vi "Handle Error.vi"(7 "Mode":T1(ring), 8 "error in (no error)":errorcluster, 9 "Test Method Name":string, 11 "Test Case Result In":refnum<class "Test Case Result.lvclass">) -> (0 "error out":errorcluster, 3 "Test Case Result Out":refnum<class "Test Case Result.lvclass">)   [LabVIEW 2020, in "Test Case Result.lvclass"]
uses:
  Test Case Result.lvclass
  Test Case Result.lvclass/Test Case Result.ctl
  Method Result/Method Result.lvclass/Method Result.ctl
  <vilib>/Utility/miscctls.llb/LVMapReplaceAction.ctl
  Method Result/Method Result.lvclass
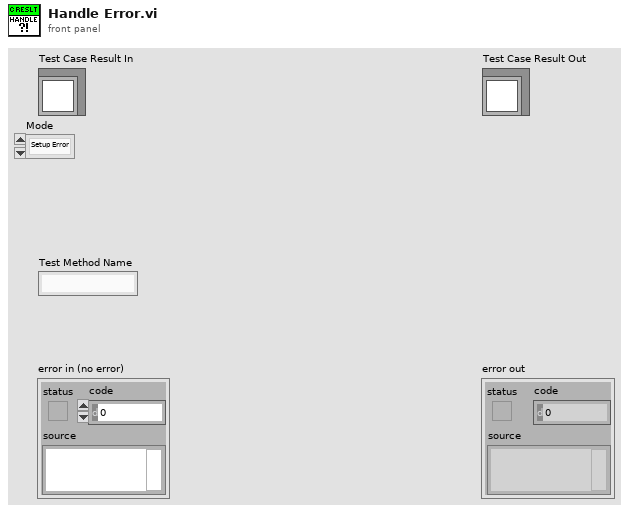
[diagram p1: front panel]
types:
  T1 = enum16{"Setup Error", "Teardown Error", "Broken", "Test Method Error"}
  T2 = typedef "LVMapReplaceAction.ctl" = enum32{"Modify Entry only if found", "Add or Modify Entry", "Delete Entry"}
  T3 = map{string, refnum<class "Method Result.lvclass">}
  T4 = typedef "Assertion Result.lvclass/Status.ctl" = enum16{"Pass", "Fail", "Error", "Skipped", "Setup Error", "Broken", "Teardown Error"}
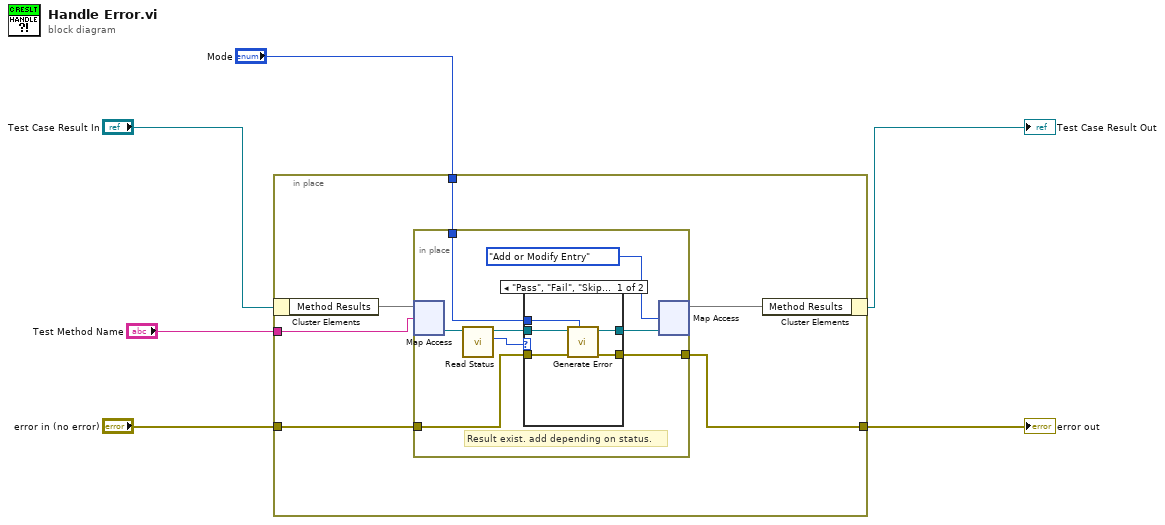
[diagram p0: block diagram]
diagram:
  n1 = in-place {
    in-place-border: "Mode" -> [w12]
    in-place-border: "error in (no error)" -> [w11]
    in-place-border: [w10] -> w4
    in-place-border: "Test Method Name" -> [w8]
    n2 = in-place-cluster #1("Test Case Result In") -> ("Method Results"=w9:T3)
    n3 = in-place {
      in-place-border: w12 -> [w16]
      in-place-border: w11 -> [w14]
      in-place-border: [w15] -> w10
      # "Result exist. add depending on status."
      n4 = in-place-map #2(w9, w8) -> (w20:refnum<class "Method Result.lvclass">)  [unwired: 1 in, 1 out]
      n5 = call "Read Status.vi"("Method Result In"=w20) -> ("Status"=w19:T4, "Method Result Out"=w18:refnum<class "Method Result.lvclass">)  [unwired: 8 in, 1 out]
      n6 = case shown="\"Pass\", \"Fail\", \"Skipped\"" w19 {
        tunnel: w18 -> [w25 w27]
        tunnel: [w24 w27] -> w17
        tunnel: w14 -> [w23 w26]
        tunnel: [w22 w26] -> w15
        tunnel: w16 -> [w21 _]
        frame "Pass", "Fail", "Skipped" {
          n7 = call "Generate Error.vi"("Mode"=w21, "error in (no error)"=w23, "Method Result In"=w25) -> ("error out"=w22:errorcluster, "Method Result Out"=w24:refnum<class "Method Result.lvclass">)  [unwired: 7 in]
        }
        frame Default {
        }
      }
      n8 = in-place-map #2(w17, LVMapReplaceAction."Add or Modify Entry" ("action")) -> (w7:T3)  [unwired: 2 out]
    }
    n9 = in-place-cluster #1("Method Results"=w7) -> (→"Test Case Result Out":refnum<class "Test Case Result.lvclass">)
  }
  "error out" <- w4
